vi "Read Messages.vi"(8 "error in":errorcluster, 11 "channel ref in":refnum<k20>) -> (0 "error out":errorcluster, 2 "messages":T1[](array[typedef]), 3 "channel ref out":refnum<k20>)   [LabVIEW 2020, in "AIM MIL-STD 1553 Import.lvlib"]
uses:
  AIM MIL-STD 1553 Import.lvlib
  dd20f27a-a9ee-486e-8ca5-fc723d32a0fb.vi
  Constants.vi
  Shared/Message Type.ctl
  Shared/Address.ctl
  Shared/Terminal Endpoint.ctl
  Shared/Parameter Definition.ctl
  Shared/Message Definition.ctl
  fd5ec535-2ba5-4254-8194-7ed8385fc538.vi
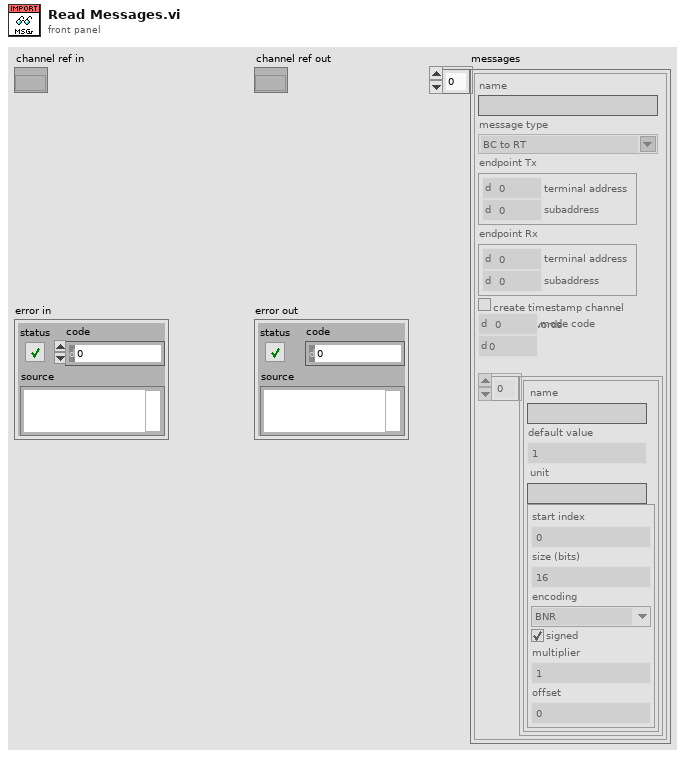
[diagram p1: front panel]
types:
  T1 = typedef "Message Definition.ctl" = cluster{"name":string, "message type":T2, "endpoint Tx":T3, "endpoint Rx":T3, "create timestamp channel":bool, "mode code":u16, "number of words":u16, "parameters":cluster{"name":string, "default value":dbl, "unit":string, "parameter definition":T5}[]}
  T2 = typedef "Message Type.ctl" = string
  T3 = typedef "Terminal Endpoint.ctl" = cluster{"terminal address":T4, "subaddress":T4}
  T4 = typedef "Address.ctl" = u16
  T5 = typedef "Parameter Definition.ctl" = cluster{"start index":i32, "size (bits)":i32, "encoding":enum16{"BNR", "BCD", "Discrete"}, "signed":bool, "multiplier":dbl, "offset":dbl}
  T6 = cluster{"name":string, "default value":dbl, "unit":string, "parameter definition":T5}[]
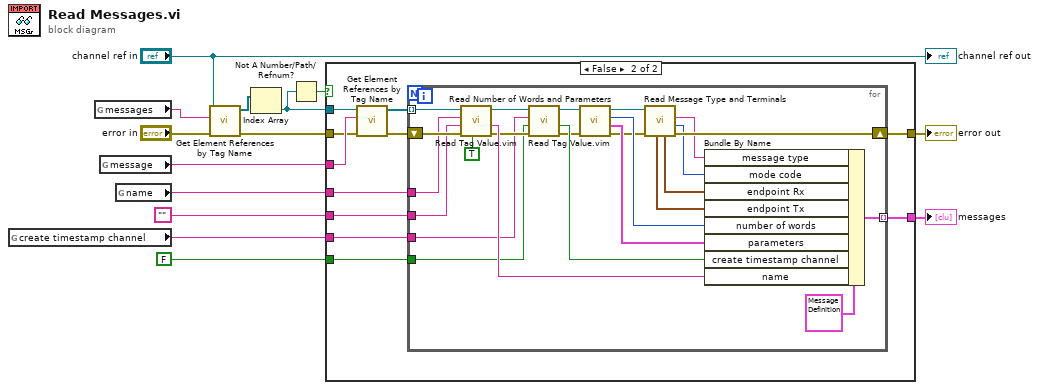
[diagram p0: block diagram]
diagram:
  n1 = global read "Constants.vi" "create timestamp channel"() -> (w9:string)
  n2 = global read "Constants.vi" "messages"() -> (w3:string)
  n3 = global read "Constants.vi" "message"() -> (w14:string)
  n4 = global read "Constants.vi" "name"() -> (w12:string)
  n5 = call "Get Element References by Tag Name.vi"("error in"="error in", "tag name"=w3, "node in"="channel ref in") -> ("error out"=w5:errorcluster, "array of elements"=w7:refnum<k20>[])  [unwired: 7 in]
  n6 = Index Array(array=w7) -> (element=w4:refnum<k20>)  [unwired: 1 in]
  n7 = Not A Number/Path/Refnum?(number/path/refnum=w4) -> (NaN/Path/Refnum?=w1:bool)
  n8 = case shown="False" w1 {
    tunnel: w14 -> [_ w26]
    tunnel: [w15 w24] -> w13
    tunnel: w12 -> [_ w22]
    tunnel: "" -> [_ w21]
    tunnel: [_ w20] -> w10
    tunnel: w9 -> [_ w19]
    tunnel: FALSE -> [_ w18]
    tunnel: w5 -> [w15 w17]
    tunnel: w4 -> [_ w16]
    frame True {
    }
    frame False {
      n9 = call "Get Element References by Tag Name.vi"("error in"=w17, "tag name"=w26, "node in"=w16) -> ("error out"=w23:errorcluster, "array of elements"=w25:refnum<k20>[])  [unwired: 7 in]
      n10 = for {
        shift-right: [w29] -> w24
        shift-left: w23 -> [w50]
        tunnel: w25 -> [w49] mode=indexing
        tunnel: w22 -> [w48]
        tunnel: w21 -> [w47]
        tunnel: [w44] -> w20 mode=indexing
        tunnel: w19 -> [w41]
        tunnel: w18 -> [w40]
        n11 = call "Read Tag Value.vim"("required (F)"=TRUE, "error in"=w50, "default"=w47, "tag name"=w48, "node in"=w49) -> ("error out"=w42:errorcluster, "value"=w45:string, "node out"=w43:refnum<k20>)  [unwired: 4 in]
        n12 = call "Read Tag Value.vim"("error in"=w42, "default"=w40, "tag name"=w41, "node in"=w43) -> ("error out"=w37:errorcluster, "value"=w39:bool, "node out"=w38:refnum<k20>)  [unwired: 5 in]
        n13 = call "Read Number of Words and Parameters.vi"("error in"=w37, "message ref in"=w38) -> ("error out"=w30:errorcluster, "parameters"=w35:T6, "number of words"=w36:u16, "message ref out"=w31:refnum<k20>)  [unwired: 6 in]
        n14 = call "Read Message Type and Terminals.vi"("error in"=w30, "message ref in"=w31) -> ("error out"=w29:errorcluster, "mode code"=w27:u16, "message type"=w28:T2, "Rx terminal"=w33:T3, "Tx terminal"=w34:T3)  [unwired: 4 in, 1 out]
        n15 = Bundle By Name(cluster=T1 {"name"="", "message type"="BC to RT", "endpoint Tx"={"terminal address"=0, "subaddress"=0}, "endpoint Rx"={"terminal address"=0, "subaddress"=0}, "create timestamp channel"=FALSE, "mode code"=0, "number of words"=0, "parameters"=[]} ("message definition"), "message type"=w28, "mode code"=w27, "endpoint Rx"=w33, "endpoint Tx"=w34, "number of words"=w36, "parameters"=w35, "create timestamp channel"=w39, "name"=w45) -> (w44:T1)
      }
    }
  }
  "error out" <- w13
  "messages" <- w10
  "channel ref out" <- "channel ref in"
